vi "M04 Smart Grid.vi"(9 "Target angle":sgl, 11 "EV3 in":T1) -> (3 "EV3 out":T1)   [LabVIEW 2016]
uses:
  <vilib>/NXT/Subs/LVHSConnector.ctl
  <vilib>/NXT/LegoClasses/BrickReference/BrickReference.lvclass
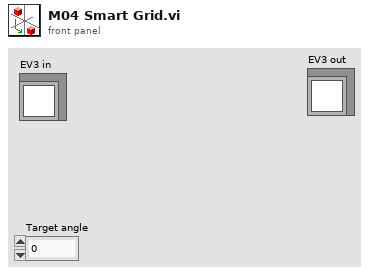
[diagram p1: front panel]
types:
  T1 = typedef "LVHSConnector.ctl" = refnum<class "BrickReference.lvclass">
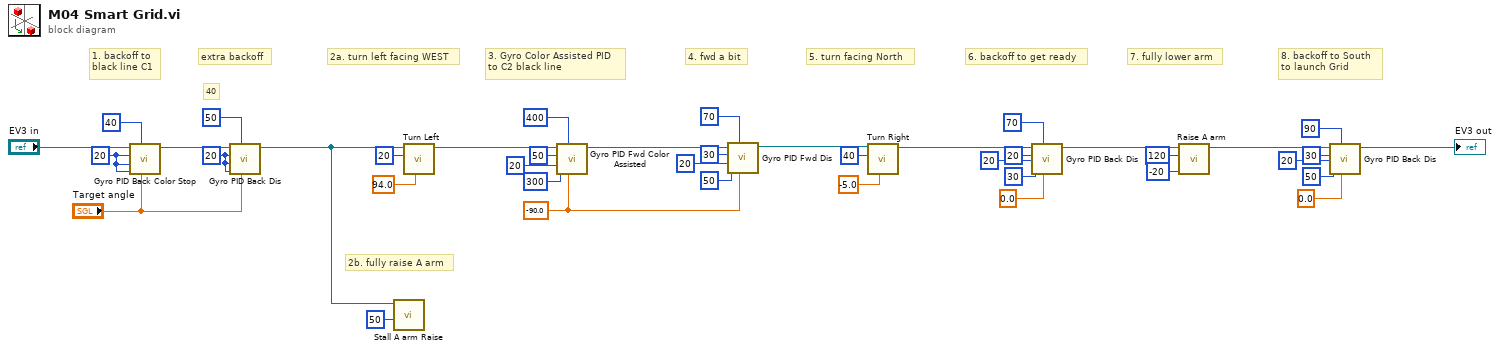
[diagram p0: block diagram]
diagram:
  w3 = 20 ("Max. speed")
  w14 = 20 ("Max. speed")
  w30 = sgl -90.0 ("Target angle")
  # "40"
  # "extra backoff"
  # "7. fully lower arm"
  # "6. backoff to get ready"
  # "2b. fully raise A arm"
  # "1. backoff to\nblack line C1"
  # "8. backoff to South\nto launch Grid"
  # "5. turn facing North"
  # "4. fwd a bit"
  # "3. Gyro Color Assisted PID\nto C2 black line"
  # "2a. turn left facing WEST"
  n1 = call "Gyro PID Back Color Stop.vi"("Target angle"="Target angle", "Threshold to Color"=40, "Threshold to slow"=w14, "Min. speed"=w14, "Max. speed"=w14, "EV3 in"="EV3 in") -> ("EV3 out"=w13:T1)  [unwired: 5 in]
  n2 = call "Gyro PID Back Dis.vi"("Target angle"="Target angle", "Threshold to stop"=50, "Threshold to slow"=w3, "Min. speed"=w3, "Max. speed"=w3, "EV3 in"=w13) -> ("EV3 out"=w5:T1)  [unwired: 5 in]
  n3 = call "Stall A arm Raise.vi"("Power"=i8 50, "NXT/EV3"=w5) -> ()  [unwired: 9 in, 1 out]
  n4 = call "Turn Left.vi"("Turning angle"=sgl 94.0, "Motor B (right)"=i8 20, "EV3 in"=w5) -> ("EV3 out"=w20:T1)  [unwired: 8 in]
  n5 = call "Gyro PID Fwd Color Assisted.vi"("Target angle"=w30, "Threshold to Color"=400, "Threshold to slow"=300, "Min. speed"=20, "Max. speed"=50, "EV3 in"=w20) -> ("EV3 out"=w35:T1)  [unwired: 5 in]
  n6 = call "Gyro PID Fwd Dis.vi"("Target angle"=w30, "Threshold to stop"=70, "Threshold to slow"=50, "Min. speed"=20, "Max. speed"=30, "EV3 in"=w35) -> ("EV3 out"=w29:T1)  [unwired: 5 in]
  n7 = call "Turn Right.vi"("Turning angle"=sgl -5.0, "Motor B (right)"=i8 40, "EV3 in"=w29) -> ("EV3 out"=w7:T1)  [unwired: 8 in]
  n8 = call "Gyro PID Back Dis.vi"("Target angle"=sgl 0.0, "Threshold to stop"=70, "Threshold to slow"=30, "Min. speed"=20, "Max. speed"=20, "EV3 in"=w7) -> ("EV3 out"=w6:T1)  [unwired: 5 in]
  n9 = call "Raise A arm.vi"("Power"=i8 -20, "Rotation"=120, "EV3 in"=w6) -> ("EV3 out"=w17:T1)  [unwired: 8 in]
  n10 = call "Gyro PID Back Dis.vi"("Target angle"=sgl 0.0, "Threshold to stop"=90, "Threshold to slow"=50, "Min. speed"=20, "Max. speed"=30, "EV3 in"=w17) -> ("EV3 out"=→"EV3 out":T1)  [unwired: 5 in]
